vi "Geometric Leaves to Objects.vi"(11 "Geometric Items":T1(array[cluster])) -> (3 "Geometric Objects":refnum<class "Geometric.lvclass">[](array[class]))   [LabVIEW 2019, in "ParseGDSII.lvclass"]
uses:
  ParseGDSII.lvclass
  Elements/Geometric.lvclass
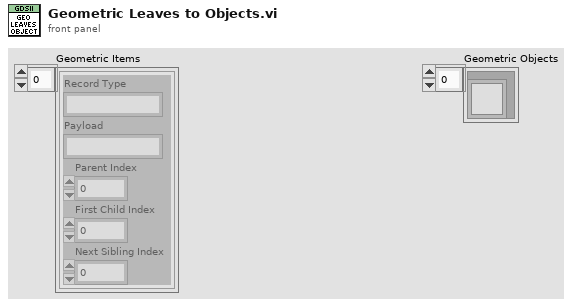
[diagram p1: front panel]
types:
  T1 = cluster{"Record Type":string, "Payload":string, "Parent Index":i32, "First Child Index":i32, "Next Sibling Index":i32}[]
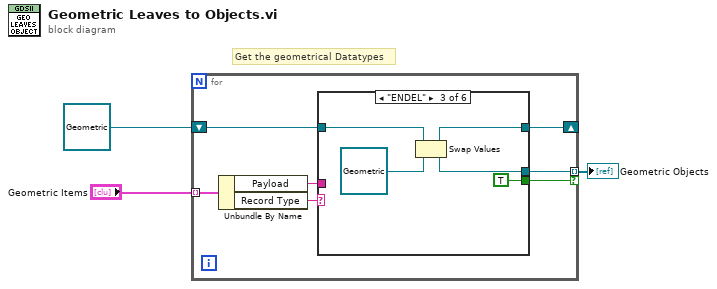
[diagram p0: block diagram]
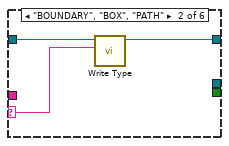
[diagram p3: hidden frame]
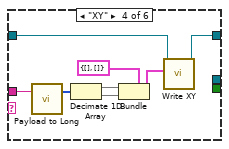
[diagram p4: hidden frame]
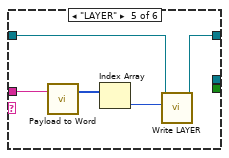
[diagram p5: hidden frame]
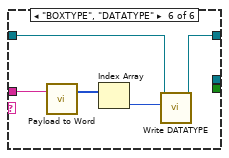
[diagram p6: hidden frame]
diagram:
  # "Get the geometrical Datatypes"
  n1 = for {
    tunnel: "Geometric Items" -> [w10] mode=indexing
    tunnel: [w5] -> w1 mode=indexing if=w4
    shift-right: [w7] -> _
    shift-left: refnum<class "Geometric.lvclass"> refnum ("Element out") -> [w6]
    n2 = Unbundle By Name(w10) -> ("Payload"=w9:string, "Record Type"=w8:string)
    n3 = case shown="\"ENDEL\"" w8 {
      selector: w8 -> [_ w12 _ _ _ _]
      tunnel: w9 -> [_ _ _ w22 w30 w36]
      tunnel: [w11 w14 w15 w21 w28 w34] -> w7
      tunnel: w6 -> [w11 w13 w16 w20 w29 w35]
      tunnel: [_ _ w17 _ _ _] -> w5
      tunnel: [_ _ TRUE _ _ _] -> w4
      frame Default {
      }
      frame "BOUNDARY", "BOX", "PATH" {
        n4 = call-dynamic "Write Type.vi"("Type"=w12, "Element in"=w13) -> ("Element out"=w14:refnum<class "Geometric.lvclass">)  [unwired: 8 in, 1 out]
      }
      frame "ENDEL" {
        n5 = Swap Values(12:w16, 14:refnum<class "Geometric.lvclass"> refnum ("Element out")) -> (1:w15:refnum<class "Geometric.lvclass">, 3:w17:refnum<class "Geometric.lvclass">)  [unwired: 1 in]
      }
      frame "XY" {
        n6 = call "Payload to Long.vi"("Payload"=w22) -> ("Long"=w25:i32[])  [unwired: 2 in]
        n7 = Decimate 1D Array(w25) -> (w27:i32[], w26:i32[])
        n8 = Bundle(cluster=cluster{"X":i32[], "Y":i32[]} {"X"=[], "Y"=[]} ("XY"), "X"=w27, "Y"=w26) -> (w24:cluster{"X":i32[], "Y":i32[]})
        n9 = call-dynamic "Write XY.vi"("XY"=w24, "Element in"=w20) -> ("Element out"=w21:refnum<class "Geometric.lvclass">)  [unwired: 8 in, 1 out]
      }
      frame "LAYER" {
        n10 = call "Payload to Word.vi"("Payload"=w30) -> ("Word"=w31:i16[])  [unwired: 2 in]
        n11 = Index Array(array=w31) -> (element=w32:i16)  [unwired: 1 in]
        n12 = call-dynamic "Write LAYER.vi"("LAYER"=w32, "Geometric in"=w29) -> ("Geometric out"=w28:refnum<class "Geometric.lvclass">)  [unwired: 8 in, 1 out]
      }
      frame "BOXTYPE", "DATATYPE" {
        n13 = call "Payload to Word.vi"("Payload"=w36) -> ("Word"=w37:i16[])  [unwired: 2 in]
        n14 = Index Array(array=w37) -> (element=w33:i16)  [unwired: 1 in]
        n15 = call-dynamic "Write DATATYPE.vi"("DATATYPE"=w33, "Geometric in"=w35) -> ("Geometric out"=w34:refnum<class "Geometric.lvclass">)  [unwired: 8 in, 1 out]
      }
    }
  }
  "Geometric Objects" <- w1
